vi "DSF.Engine.Transceiver.Shutdown.vi"(8 "error in (no error)":errorcluster, 11 "Transceiver in":refnum<class "DSF.Engine.Transceiver.lvclass">) -> (0 "error out":errorcluster, 3 "Transceiver out":refnum<class "DSF.Engine.Transceiver.lvclass">)   [LabVIEW 2017, in "DSF.Engine.lvlib" / "DSF.Engine.Transceiver.lvclass"]
uses:
  DSF.Engine.Transceiver.lvclass
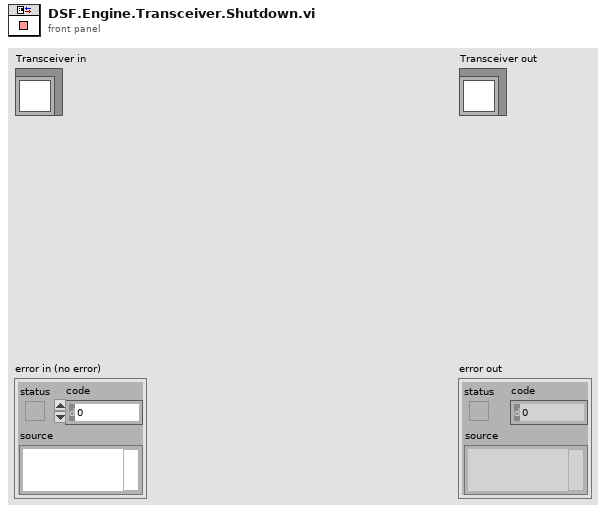
[diagram p1: front panel]
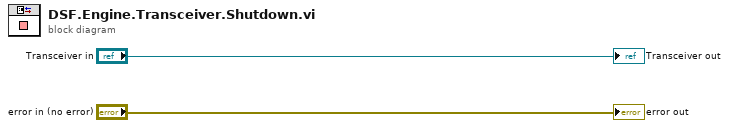
[diagram p0: block diagram]
diagram:
  "error out" <- "error in (no error)"
  "Transceiver out" <- "Transceiver in"
